vi "Begin.vi"(8 "error in":errorcluster) -> (0 "error out":errorcluster)   [LabVIEW 2017]
doc: "Called before other user functions, this VI is expected to open initial I/O refnums, load in file data, and do all program initialization. Notice that the <B>error out</B> terminal is simply used for data flow. Wiring it to other structures or subVIs ensures that this VI runs first."
uses:
  <vilib>/Rock Robotics/WPI/DriverStation/WPI_DriverStationRobotMode2.ctl
  <vilib>/Rock Robotics/WPI/Joystick/WPI_JoystickDeviceEnum.ctl
  <vilib>/Rock Robotics/WPI/Solenoid/WPI_SolenoidChannel.ctl
  <vilib>/Rock Robotics/SystemInterfaces/DIO/FPGA_DIOPWMChannel.ctl
  <vilib>/Rock Robotics/SystemInterfaces/DIO/FPGA_DIOChannel.ctl
  Robot Global Data.vi
  <vilib>/Rock Robotics/WPI/Solenoid/WPI_SolenoidOpenDouble.vi
  <vilib>/Rock Robotics/WPI/MotorControl/WPI_MotorControlOpen Talon.vi
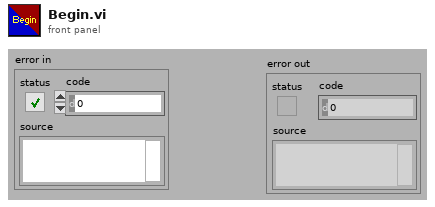
[diagram p1: front panel]
types:
  T1 = typedef "FPGA_DIOChannel.ctl" = enum8{"DIO 0", "DIO 1", "DIO 2", "DIO 3", "DIO 4", "DIO 5", "DIO 6", "DIO 7", "DIO 8", "DIO 9", "DIO MXP 0", "DIO MXP 1", "DIO MXP 2", "DIO MXP 3", "DIO MXP 4", "DIO MXP 5", "DIO MXP 6", "DIO MXP 7", "DIO MXP 8", "DIO MXP 9", "DIO MXP 10", "DIO MXP 11", "DIO MXP 12", "DIO MXP 13", "DIO MXP 14", "DIO MXP 15", "SPI Port CS1", "SPI Port CS2", "SPI Port CS3", "SPI Port MISO", "SPI Port MOSI", "Invalid"}
  T2 = typedef "WPI_JoystickDeviceEnum.ctl" = enum16{"USB 0", "USB 1", "USB 2", "USB 3", "USB 4", "USB 5"}
  T3 = typedef "FPGA_DIOPWMChannel.ctl" = enum8{"PWM 0", "PWM 1", "PWM 2", "PWM 3", "PWM 4", "PWM 5", "PWM 6", "PWM 7", "PWM 8", "PWM 9", "PWM MXP 0", "PWM MXP 1", "PWM MXP 2", "PWM MXP 3", "PWM MXP 4", "PWM MXP 5", "PWM MXP 6", "PWM MXP 7", "PWM MXP 8", "PWM MXP 9", "Invalid"}
  T4 = typedef "WPI_SolenoidChannel.ctl" = enum8{"Solenoid 0", "Solenoid 1", "Solenoid 2", "Solenoid 3", "Solenoid 4", "Solenoid 5", "Solenoid 6", "Solenoid 7", "Invalid"}
  T5 = typedef "WPI_DriverStationRobotMode2.ctl" = enum16{"Autonomous Disabled", "Autonomous Enabled", "Teleop Disabled", "Teleop Enabled", "Disconnected", "Finish", "Test Disabled", "Test Enabled", "Emergency Stopped"}
  T6 = typedef "WPI_JoystickDevRef.ctl" = cluster{"Device":T2}
  T7 = typedef "WPI_DigitalInputDevRef.ctl" = cluster{"DevStatus":errorcluster, "DIO Channel":T1}
  T8 = typedef "WPI_MotorControlDeviceRef.ctl" = cluster{"DeviceStatus":errorcluster, "Type":T9, "PWM":cluster{"PWM Channel":T3, "DeadBand":T10}, "CAN":cluster{"Device Number":u8, "SetOutput VI Ref":variant, "GetOutput VI Ref":variant, "Enable VI Ref":variant, "Disable VI Ref":variant, "Data":variant}, "Invert":bool, "DIO PWM":cluster{"PWM \"Enable\" Channel":T3, "DIOChannel":T1, "PWM Rate":dbl}}
  T9 = typedef "WPI_MotorControlType.ctl" = enum16{"PWM", "CAN", "DIO PWM"}
  T10 = typedef "WPI_PWMDeadband.ctl" = cluster{"Name":string, "maxPositivePwm":i32, "minPositivePwm":i32, "centerPwm":i32, "maxNegativePwm":i32, "minNegativePwm":i32, "angularRange":u16}
  T11 = typedef "WPI_SolenoidDevRef.ctl" = cluster{"DevStatus":errorcluster, "Pneumatics Control Module":u8, "Forward Solenoid Channel":T4, "Reverse Solenoid Channel":T4}
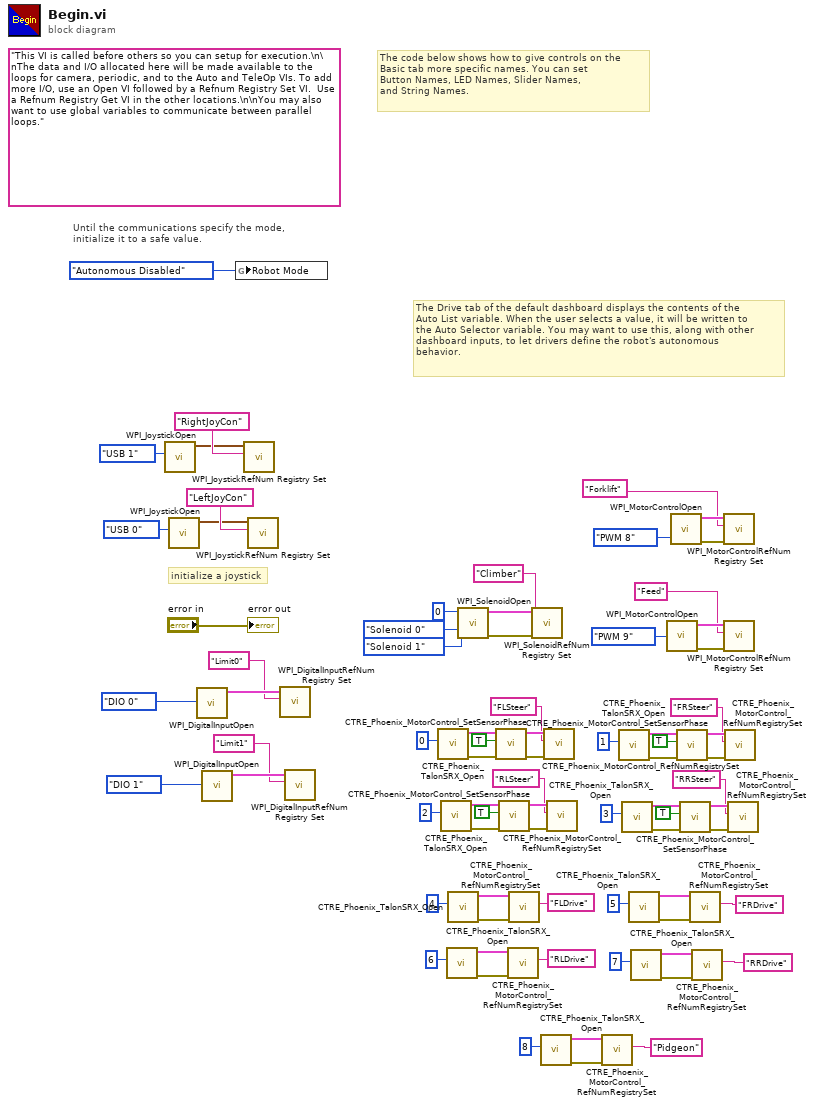
[diagram p0: block diagram]
diagram:
  (unwired) "This VI is called before others so you can setup for execution.\n\nThe data and I/O allocated here will be made available to the loops for camera, periodic, and to the Auto and TeleOp VIs. To add more I/O, use an Open VI followed by a Refnum Registry Set VI.  Use a Refnum Registry Get VI in the other locations.\n\nYou may also want to use global variables to communicate between parallel loops."
  # "The Drive tab of the default dashboard displays the contents of the\nAuto List variable. When the user selects a value, it will be written to\nthe Auto Selector variable. You may want to use this, along with other\ndashboard inputs, to let drivers define the robot's autonomous\nbehavior."
  # "The code below shows how to give controls on the\nBasic tab more specific names. You can set\nButton Names, LED Names, Slider Names,\nand String Names."
  # "initialize a joystick"
  # "Until the communications specify the mode,\ninitialize it to a safe value."
  n1 = call <vilib>:"WPI_JoystickOpen.vi"("JoystickDevice"=WPI_JoystickDeviceEnum."USB 1") -> ("JoystickDevRef"=w56:T6)  [unwired: 10 in]
  n2 = call <vilib>:"WPI_JoystickOpen.vi"("JoystickDevice"=WPI_JoystickDeviceEnum."USB 0") -> ("JoystickDevRef"=w74:T6)  [unwired: 10 in]
  n3 = call <vilib>:"WPI_DigitalInputOpen.vi"("DIO Channel"=FPGA_DIOChannel."DIO 0") -> ("DigitalInputDevRef"=w54:T7)  [unwired: 9 in, 1 out]
  n4 = call <vilib>:"WPI_DigitalInputOpen.vi"("DIO Channel"=FPGA_DIOChannel."DIO 1") -> ("DigitalInputDevRef"=w51:T7)  [unwired: 9 in, 1 out]
  n5 = global write "Robot Global Data.vi" "Robot Mode"(WPI_DriverStationRobotMode2."Autonomous Disabled" ("Robot Mode")) -> ()
  n6 = call <vilib>:"WPI_JoystickRefNum Registry Set.vi"("refnum name"="RightJoyCon", "JoystickDevRef"=w56) -> ()  [unwired: 8 in, 2 out]
  n7 = call <vilib>:"WPI_JoystickRefNum Registry Set.vi"("refnum name"="LeftJoyCon", "JoystickDevRef"=w74) -> ()  [unwired: 8 in, 2 out]
  n8 = call <vilib>:"WPI_DigitalInputRefNum Registry Set.vi"("refnum name"="Limit0", "DigitalInputDevRef"=w54) -> ()  [unwired: 8 in, 2 out]
  n9 = call <vilib>:"WPI_DigitalInputRefNum Registry Set.vi"("refnum name"="Limit1", "DigitalInputDevRef"=w51) -> ()  [unwired: 8 in, 2 out]
  n10 = call <vilib>:"CTRE_Phoenix_TalonSRX_Open.vi"("Device Number"=u8 0) -> ("error out"=w46:errorcluster, "CAN Talon SRX Ref"=w47:T8)  [unwired: 9 in]
  n11 = call <vilib>:"CTRE_Phoenix_TalonSRX_Open.vi"("Device Number"=u8 2) -> ("error out"=w39:errorcluster, "CAN Talon SRX Ref"=w40:T8)  [unwired: 9 in]
  n12 = call <vilib>:"CTRE_Phoenix_TalonSRX_Open.vi"("Device Number"=u8 6) -> ("error out"=w9:errorcluster, "CAN Talon SRX Ref"=w10:T8)  [unwired: 9 in]
  n13 = call <vilib>:"CTRE_Phoenix_TalonSRX_Open.vi"("Device Number"=u8 4) -> ("error out"=w17:errorcluster, "CAN Talon SRX Ref"=w18:T8)  [unwired: 9 in]
  n14 = call-poly <vilib>:"WPI_SolenoidOpen.vi"("Reverse Solenoid Channel"=WPI_SolenoidChannel."Solenoid 1", "Forward Solenoid Channel"=WPI_SolenoidChannel."Solenoid 0", "Pneumatics Control Module (0)"=u8 0) -> ("error out"=w66:errorcluster, "SolenoidDevRef"=w68:T11)  [unwired: 7 in]
  n15 = call <vilib>:"CTRE_Phoenix_MotorControl_SetSensorPhase.vi"("error in (no error)"=w46, "PhaseSensor"=TRUE, "PhoenixMotorControlDevRef"=w47) -> ("error out"=w44:errorcluster, "PhoenixMotorControlDevRef"=w43:T8)  [unwired: 7 in]
  n16 = call <vilib>:"CTRE_Phoenix_MotorControl_SetSensorPhase.vi"("error in (no error)"=w39, "PhaseSensor"=TRUE, "PhoenixMotorControlDevRef"=w40) -> ("error out"=w37:errorcluster, "PhoenixMotorControlDevRef"=w36:T8)  [unwired: 7 in]
  n17 = call <vilib>:"CTRE_Phoenix_MotorControl_RefNumRegistrySet.vi"("error in (no error)"=w9, "refnum name"="RLDrive", "PhoenixMotorControlDevRef"=w10) -> ()  [unwired: 7 in, 2 out]
  n18 = call <vilib>:"CTRE_Phoenix_MotorControl_RefNumRegistrySet.vi"("error in (no error)"=w17, "refnum name"="FLDrive", "PhoenixMotorControlDevRef"=w18) -> ()  [unwired: 7 in, 2 out]
  n19 = call <vilib>:"WPI_SolenoidRefNum Registry Set.vi"("error in (no error)"=w66, "refnum name"="Climber", "SolenoidDevRef"=w68) -> ()  [unwired: 7 in, 2 out]
  n20 = call <vilib>:"CTRE_Phoenix_TalonSRX_Open.vi"("Device Number"=u8 8) -> ("error out"=w1:errorcluster, "CAN Talon SRX Ref"=w2:T8)  [unwired: 9 in]
  n21 = call <vilib>:"CTRE_Phoenix_MotorControl_RefNumRegistrySet.vi"("error in (no error)"=w44, "refnum name"="FLSteer", "PhoenixMotorControlDevRef"=w43) -> ()  [unwired: 7 in, 2 out]
  n22 = call <vilib>:"CTRE_Phoenix_MotorControl_RefNumRegistrySet.vi"("error in (no error)"=w37, "refnum name"="RLSteer", "PhoenixMotorControlDevRef"=w36) -> ()  [unwired: 7 in, 2 out]
  n23 = call <vilib>:"CTRE_Phoenix_MotorControl_RefNumRegistrySet.vi"("error in (no error)"=w1, "refnum name"="Pidgeon", "PhoenixMotorControlDevRef"=w2) -> ()  [unwired: 7 in, 2 out]
  n24 = call <vilib>:"CTRE_Phoenix_TalonSRX_Open.vi"("Device Number"=u8 1) -> ("error out"=w32:errorcluster, "CAN Talon SRX Ref"=w33:T8)  [unwired: 9 in]
  n25 = call <vilib>:"CTRE_Phoenix_TalonSRX_Open.vi"("Device Number"=u8 3) -> ("error out"=w25:errorcluster, "CAN Talon SRX Ref"=w26:T8)  [unwired: 9 in]
  n26 = call <vilib>:"CTRE_Phoenix_TalonSRX_Open.vi"("Device Number"=u8 5) -> ("error out"=w13:errorcluster, "CAN Talon SRX Ref"=w14:T8)  [unwired: 9 in]
  n27 = call <vilib>:"CTRE_Phoenix_TalonSRX_Open.vi"("Device Number"=u8 7) -> ("error out"=w5:errorcluster, "CAN Talon SRX Ref"=w6:T8)  [unwired: 9 in]
  n28 = call-poly <vilib>:"WPI_MotorControlOpen.vi"("PWM Channel"=FPGA_DIOPWMChannel."PWM 9") -> ("error out"=w61:errorcluster, "MotorControlDeviceRef"=w60:T8)  [unwired: 9 in]
  n29 = call-poly <vilib>:"WPI_MotorControlOpen.vi"("PWM Channel"=FPGA_DIOPWMChannel."PWM 8") -> ("error out"=w64:errorcluster, "MotorControlDeviceRef"=w65:T8)  [unwired: 9 in]
  n30 = call <vilib>:"CTRE_Phoenix_MotorControl_SetSensorPhase.vi"("error in (no error)"=w32, "PhaseSensor"=TRUE, "PhoenixMotorControlDevRef"=w33) -> ("error out"=w30:errorcluster, "PhoenixMotorControlDevRef"=w29:T8)  [unwired: 7 in]
  n31 = call <vilib>:"CTRE_Phoenix_MotorControl_SetSensorPhase.vi"("error in (no error)"=w25, "PhaseSensor"=TRUE, "PhoenixMotorControlDevRef"=w26) -> ("error out"=w23:errorcluster, "PhoenixMotorControlDevRef"=w22:T8)  [unwired: 7 in]
  n32 = call <vilib>:"CTRE_Phoenix_MotorControl_RefNumRegistrySet.vi"("error in (no error)"=w13, "refnum name"="FRDrive", "PhoenixMotorControlDevRef"=w14) -> ()  [unwired: 7 in, 2 out]
  n33 = call <vilib>:"CTRE_Phoenix_MotorControl_RefNumRegistrySet.vi"("error in (no error)"=w5, "refnum name"="RRDrive", "PhoenixMotorControlDevRef"=w6) -> ()  [unwired: 7 in, 2 out]
  n34 = call <vilib>:"WPI_MotorControlRefNum Registry Set.vi"("error in (no error)"=w64, "refnum name"="Forklift", "MotorControlDevRef"=w65) -> ()  [unwired: 7 in, 2 out]
  n35 = call <vilib>:"WPI_MotorControlRefNum Registry Set.vi"("error in (no error)"=w61, "refnum name"="Feed", "MotorControlDevRef"=w60) -> ()  [unwired: 7 in, 2 out]
  n36 = call <vilib>:"CTRE_Phoenix_MotorControl_RefNumRegistrySet.vi"("error in (no error)"=w30, "refnum name"="FRSteer", "PhoenixMotorControlDevRef"=w29) -> ()  [unwired: 7 in, 2 out]
  n37 = call <vilib>:"CTRE_Phoenix_MotorControl_RefNumRegistrySet.vi"("error in (no error)"=w23, "refnum name"="RRSteer", "PhoenixMotorControlDevRef"=w22) -> ()  [unwired: 7 in, 2 out]
  "error out" <- "error in"
